vi "IMAQdx Acquisition Template (Host)RT-8output.vi"() -> ()   [LabVIEW 2016]
uses:
  <vilib>/userdefined/High Color/IMAQdx.ctl
  <vilib>/FPGAPlugInAG/roboRIO/niLvFpga_Open_roboRIO.vi
  <vilib>/rvi/interface/common/dynamic/niFpgaDynamicAddResources.vi
  <vilib>/FPGAPlugInAG/Dynamic/niLvFpga_Download_Dynamic.vi
  <vilib>/FPGAPlugInAG/Dynamic/niLvFpga_Run_Dynamic.vi
  <vilib>/Utility/error.llb/Error Cluster From Error Code.vi
  <vilib>/rvi/errors/niLvFpgaAdjustHostInterfaceError.vi
  <vilib>/rvi/interface/common/niFpgaWaitOnOcc.vi
  <vilib>/vision/EDVR.llb/IMAQ ImageToEDVR 2D U32.vi
  <vilib>/FPGAPlugInAG/Dynamic/niLvFpga_Close_Dynamic.vi
  <vilib>/rvi/interface/nirviOpenFPGA/nirviOpenFPGA.xnode
  FPGA Bitfiles/ImageProcessingw_FPGATarget_ImageProcessingw_Z23Lc7CsNwk.lvbitx
  <vilib>/rvi/interface/nirviMethod/nirviMethod.xnode
  <vilib>/rvi/interface/nirviReadWriteControl/nirviReadWriteControl.xnode
  <vilib>/rvi/interface/nirviCloseFPGA/nirviCloseFPGA.xnode
  <vilib>/vision/driver/NI_Vision_Acquisition_Software.lvlib
  <resource>/objmgr/imaqdx.rc
  <vilib>/rvi/interface/Simulation/niFpgaSimulationCallBeginRW.vi
  <vilib>/rvi/errors/niLvFpgaMergeErrorWithErrorCode.vi
  <vilib>/FPGAPlugInAG/Dynamic/niLvFpga_ReadFifo_Dynamic.vi
  <vilib>/FPGAPlugInAG/Dynamic/niLvFpga_ConfigureFifo_Dynamic.vi
  <vilib>/FPGAPlugInAG/Dynamic/niLvFpga_StartFifo_Dynamic.vi
  NiFpgaLv.dll
  <vilib>/FPGAPlugInAG/Dynamic/niLvFpga_WriteFifo_Dynamic.vi
panel:
  out "RecGaussian2?":bool
  out "RecGaussian1?":bool
  out "Error Out 2":errorcluster
  in  "Stop":bool
  in  "Maximum Pixels per Write":u32=261244
  out "dePixelCount":u32
  out "AllPixelCount":u32
  out "error out 2":errorcluster
  in  "Camera":T1="cam0"
  # "Overview: Demonstrates how to acquire an image from a camera using the IMAQdx API, transfer the image to a FPGA target for processing, and retrieve the processed image for display or further processing on the host.\nRequirements:\n- LabVIEW FPGA\n- Vision Acquisition Software\n- Vision Development Module\nInstructions:\n1. Select a Camera\n2. Run the VI."
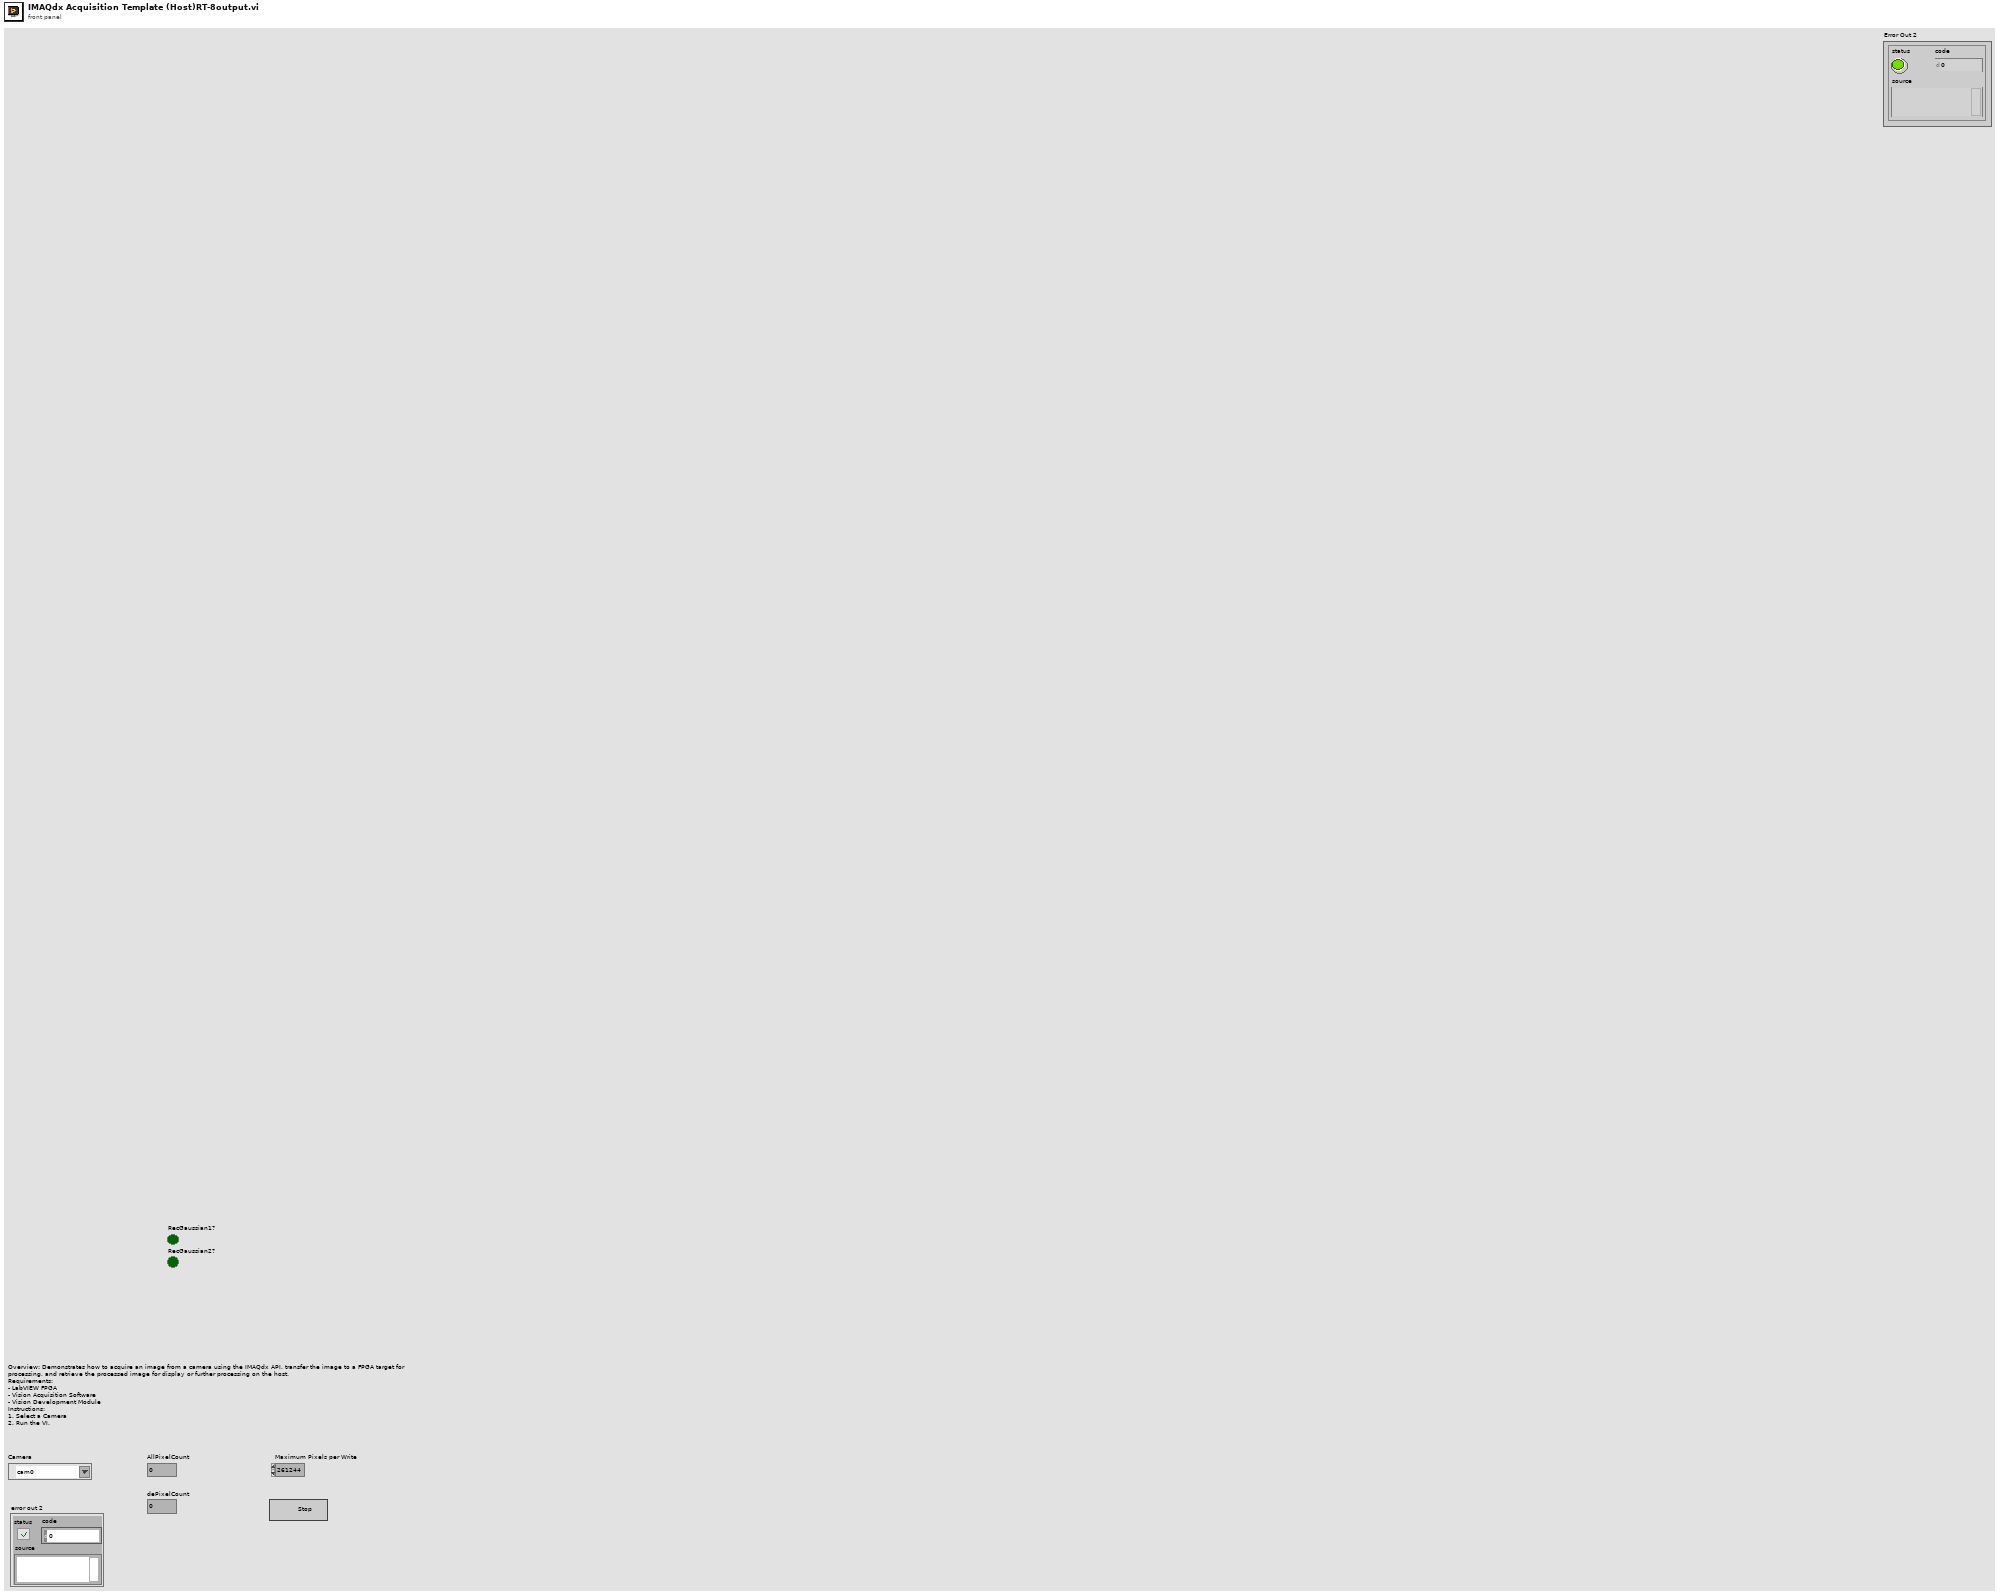
[diagram p1: front panel]
types:
  T1 = typedef "IMAQdx.ctl" = refnum<k21>
  T2 = typedef "Image Type" = u32
  T3 = typedef "IMAQ Image.ctl" = refnum<image>
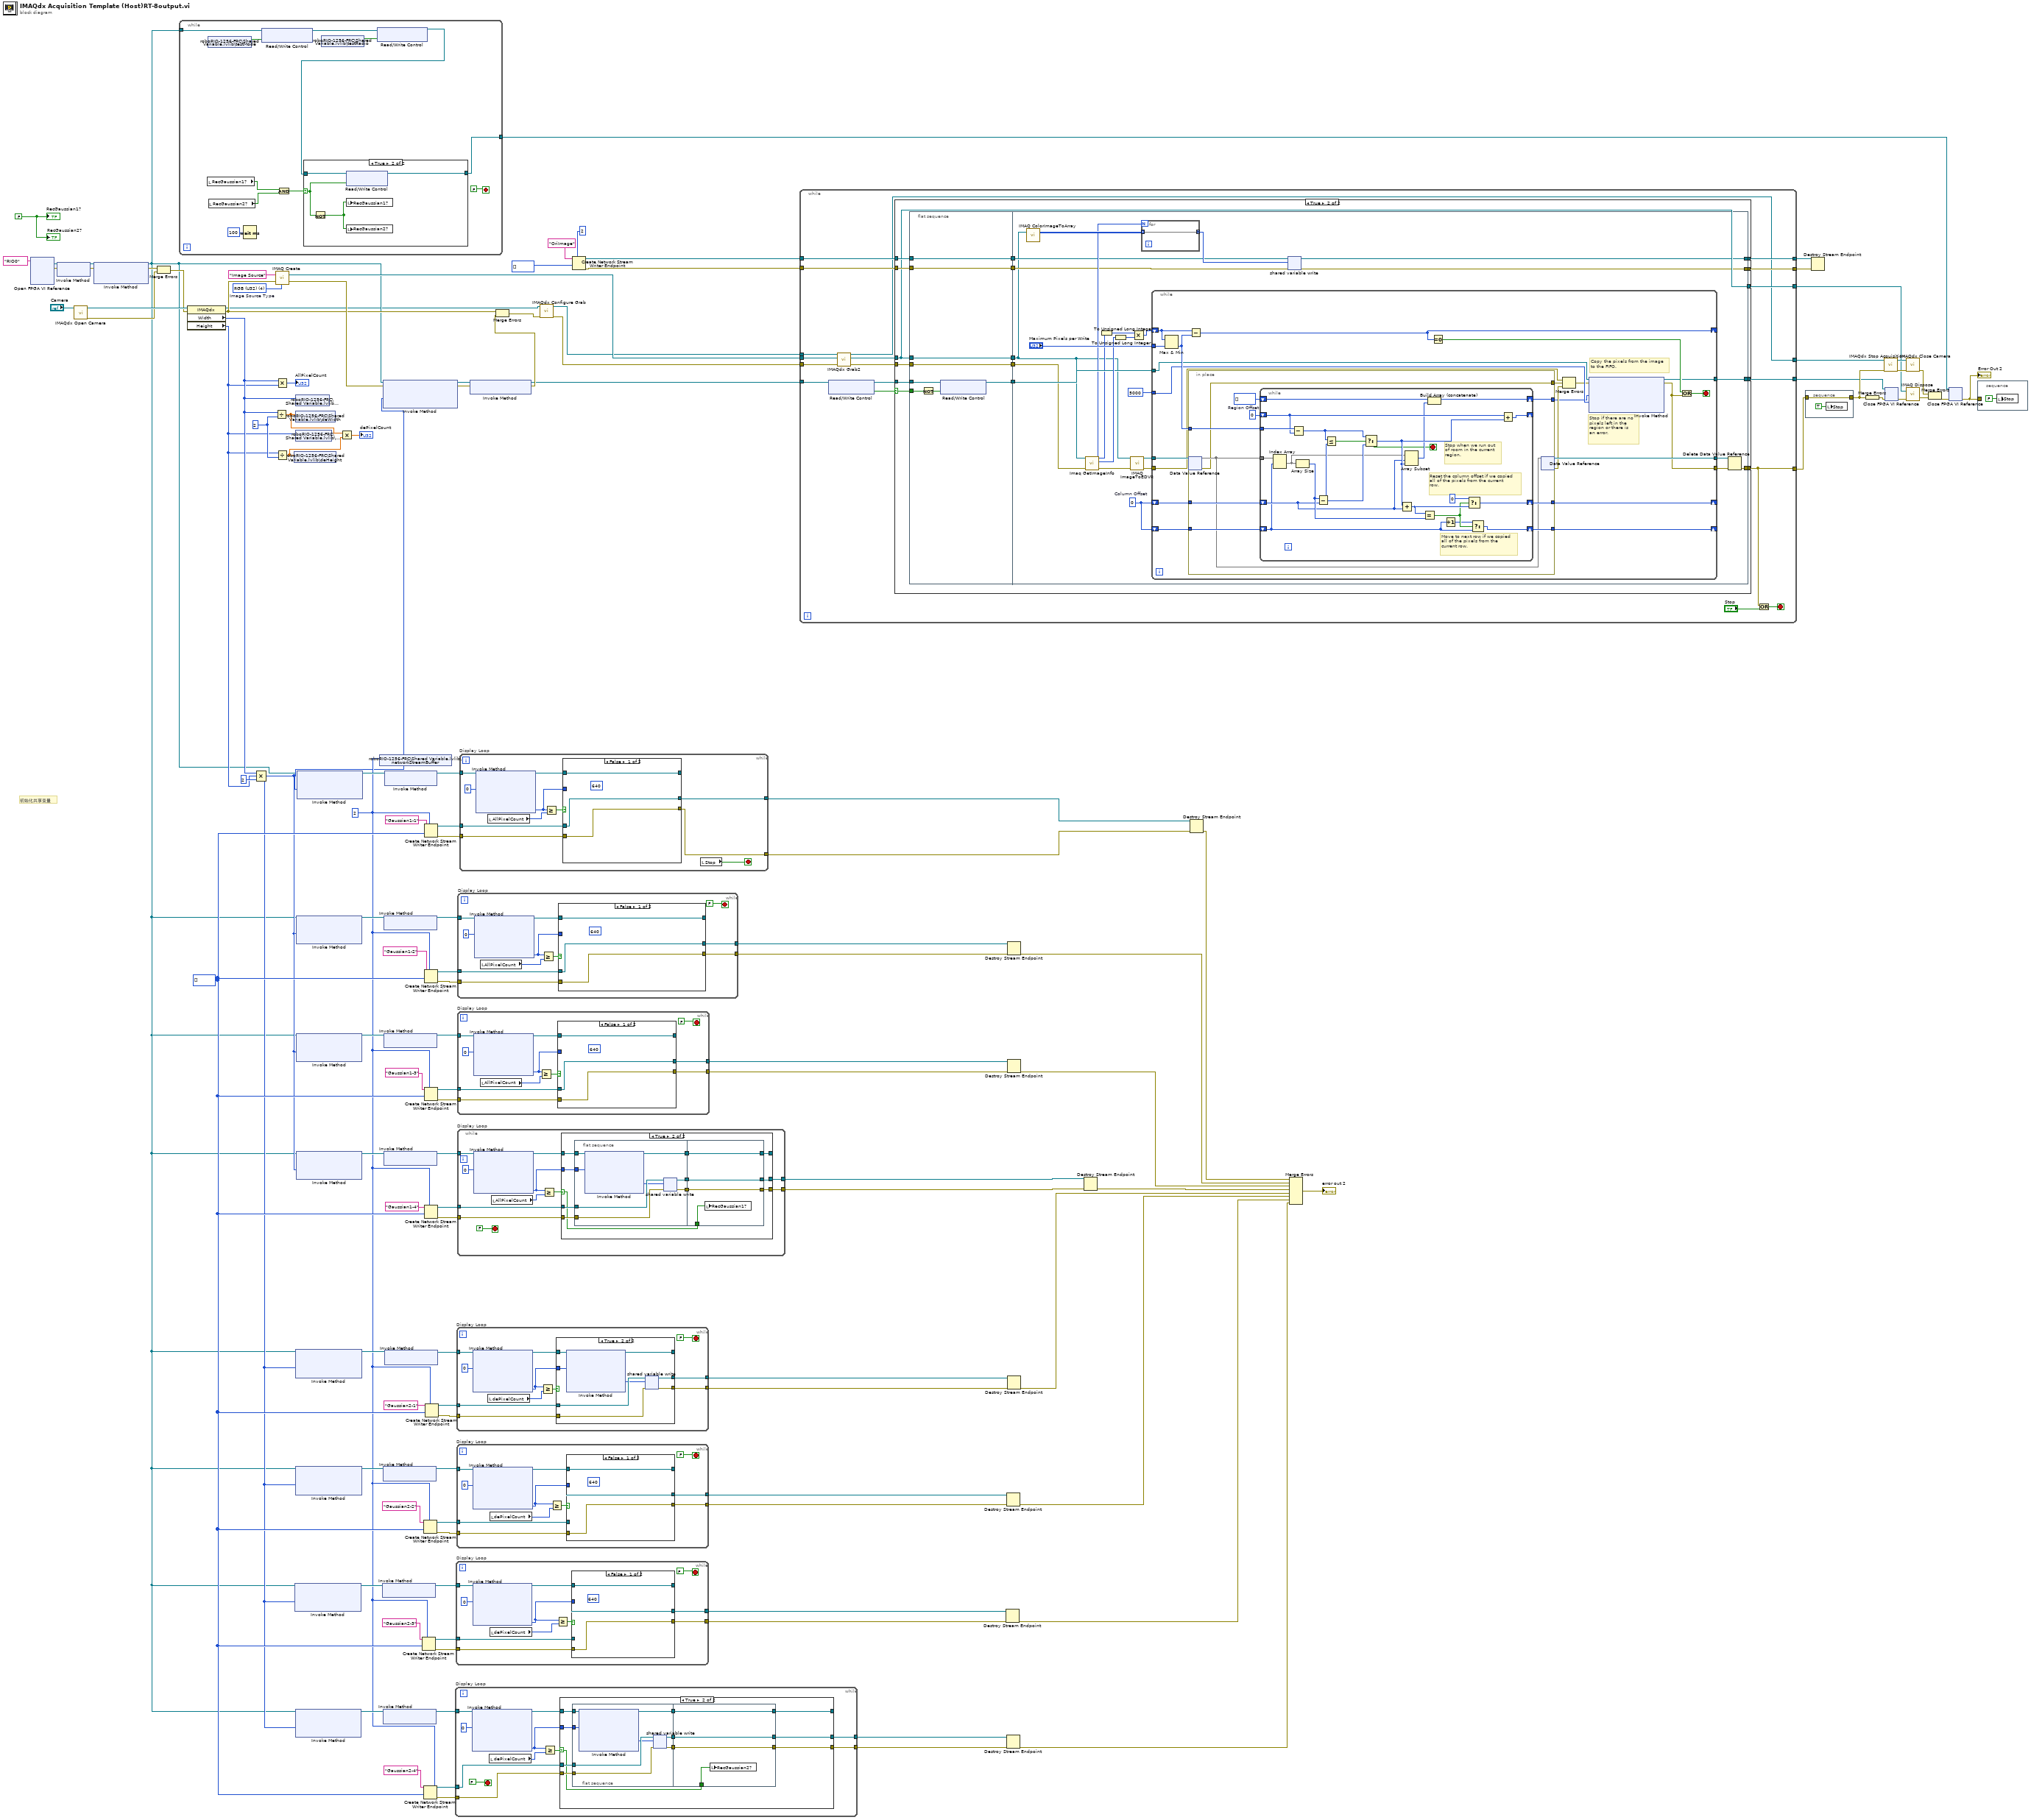
[diagram p0: block diagram]
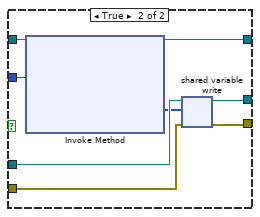
[diagram p4: hidden frame]
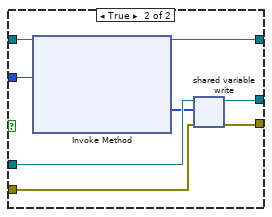
[diagram p5: hidden frame]
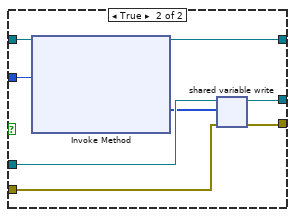
[diagram p9: hidden frame]
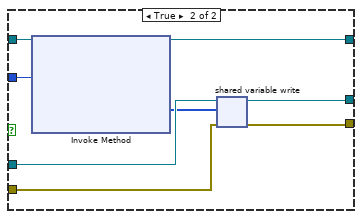
[diagram p10: hidden frame]
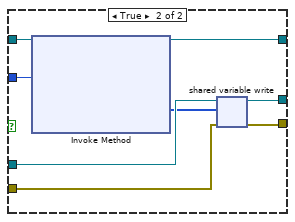
[diagram p11: hidden frame]
diagram:
  w1 = FALSE
  w42 = u32 2 ("y")
  w51 = i32[] []
  w48 = 2 ("writer buffer size")
  w111 = T2 4 items=["Grayscale (U8)", "Grayscale (I16)", "Grayscale (SGL)", "Complex (CSG)", "RGB (U32)", "HSL (U32)", "RGB (U64)", "Grayscale (U16)"]  # Image Source Type
  # "初始化共享变量"
  n1 = xnode "Open FPGA VI Reference"("resource name"=tag "RIO0") -> ("FPGA VI Reference Out"=w118:refnum<k20>, "error out"=w119:errorcluster)  [unwired: 1 in]
  n2 = xnode "Invoke Method"("FPGA VI Reference In"=w118, "error in"=w119) -> ("FPGA VI Reference Out"=w121:refnum<k20>, "error out"=w120:errorcluster)
  n3 = call <vilib>:"IMAQdx Open Camera.vi"("Session In"="Camera") -> ("error out"=w113:errorcluster, "Session Out"=w114:T1)  [unwired: 9 in]
  n4 = xnode "Invoke Method"("FPGA VI Reference In"=w121, "error in"=w120) -> ("FPGA VI Reference Out"=w6:refnum<k20>, "error out"=w115:errorcluster)  [unwired: 1 in]
  n5 = Merge Errors(w115, w113) -> (w112:errorcluster)
  n6 = while {
    tunnel: w6 -> [w128]
    tunnel: [w123] -> w9
    stop <- FALSE stop-if-true
    n7 = local read "RecGaussian1?"() -> (w132:bool)
    n8 = shared-variable "roboRIO-1256-FRC\\Shared Variable.lvlib\\testMode"() -> (w127:bool)  [unwired: 1 in, 1 out]
    n9 = local read "RecGaussian2?"() -> (w131:bool)
    n10 = Wait (ms)(milliseconds to wait=u32 100) -> ()  [unwired: 1 out]
    n11 = xnode "Read/Write Control"("FPGA VI Reference In"=w128, "Mode LED Status"=w127) -> ("FPGA VI Reference Out"=w126:refnum<k20>)  [unwired: 1 in, 1 out]
    n12 = And(x=w132, y=w131) -> (x .and. y?=w130:bool)
    n13 = shared-variable "roboRIO-1256-FRC\\Shared Variable.lvlib\\testRadio"() -> (w125:bool)  [unwired: 1 in, 1 out]
    n14 = xnode "Read/Write Control"("FPGA VI Reference In"=w126, "Radio LED Status"=w125) -> ("FPGA VI Reference Out"=w124:refnum<k20>)  [unwired: 1 in, 1 out]
    n15 = case shown="True" w130 {
      selector: w130 -> [_ w136]
      tunnel: w124 -> [w134 w138]
      tunnel: [w134 w137] -> w123
      frame False {
      }
      frame True {
        n16 = Not(x=w136) -> (.not. x?=w135:bool)
        n17 = xnode "Read/Write Control"("FPGA VI Reference In"=w138, "StartOfImage"=w136) -> ("FPGA VI Reference Out"=w137:refnum<k20>)  [unwired: 1 in, 1 out]
        n18 = local write "RecGaussian1?"(w135) -> ()
        n19 = local write "RecGaussian2?"(w135) -> ()
      }
    }
  }
  n20 = property class="IMAQdx"(reference=w114, error in=w112) -> (reference out=w5:T1, error out=w31:errorcluster, "Width"=w41:u32, "Height"=w40:u32)
  n21 = Compound Arithmetic op=MULTIPLY(w41, w40, u32 2 ("value")) -> (w35:u32)
  n22 = Divide(x=w41, y=w42) -> (x/y=w37:dbl)
  n23 = call "IMAQ Create"("Image Name"="Image Source", "Image Type"=w111, "error in (no error)"=w31) -> ("New Image"=w7:T3, "error out"=w34:errorcluster)  [unwired: 2 in]
  n24 = Multiply(x=w41, y=w40) -> (x*y=→"AllPixelCount":u32)
  n25 = Divide(x=w40, y=w42) -> (x/y=w36:dbl)
  n26 = shared-variable "roboRIO-1256-FRC\\Shared Variable.lvlib\\deHeight"(w36) -> ()  [unwired: 1 in, 1 out]
  n27 = xnode "Invoke Method"("FPGA VI Reference In"=w6, "Requested Depth"=w35) -> ("FPGA VI Reference Out"=w56:refnum<k20>)  [unwired: 1 in, 2 out]
  n28 = shared-variable "roboRIO-1256-FRC\\Shared Variable.lvlib\\Width"(w41) -> ()  [unwired: 1 in, 1 out]
  n29 = shared-variable "roboRIO-1256-FRC\\Shared Variable.lvlib\\deWidth"(w37) -> ()  [unwired: 1 in, 1 out]
  n30 = xnode "Invoke Method"("FPGA VI Reference In"=w6, "Requested Depth"=w35) -> ("FPGA VI Reference Out"=w79:refnum<k20>)  [unwired: 1 in, 2 out]
  n31 = shared-variable "roboRIO-1256-FRC\\Shared Variable.lvlib\\Height"(w40) -> ()  [unwired: 1 in, 1 out]
  n32 = xnode "Invoke Method"("FPGA VI Reference In"=w6, "Requested Depth"=w35) -> ("FPGA VI Reference Out"=w50:refnum<k20>)  [unwired: 1 in, 2 out]
  n33 = xnode "Invoke Method"("FPGA VI Reference In"=w6, "Requested Depth"=w35) -> ("FPGA VI Reference Out"=w61:refnum<k20>)  [unwired: 1 in, 2 out]
  n34 = xnode "Invoke Method"("FPGA VI Reference In"=w6, "Requested Depth"=w35) -> ("FPGA VI Reference Out"=w94:refnum<k20>)  [unwired: 1 in, 2 out]
  n35 = xnode "Invoke Method"("FPGA VI Reference In"=w6, "Requested Depth"=w35) -> ("FPGA VI Reference Out"=w91:refnum<k20>)  [unwired: 1 in, 2 out]
  n36 = xnode "Invoke Method"("FPGA VI Reference In"=w6, "Requested Depth"=w35) -> ("FPGA VI Reference Out"=w73:refnum<k20>)  [unwired: 1 in, 2 out]
  n37 = xnode "Invoke Method"("FPGA VI Reference In"=w6, "Requested Depth"=w35) -> ("FPGA VI Reference Out"=w110:refnum<k20>)  [unwired: 1 in, 2 out]
  n38 = Multiply(x=w37, y=w36) -> (x*y=→"dePixelCount":dbl)
  n39 = shared-variable "roboRIO-1256-FRC\\Shared Variable.lvlib\\networkStreamBuffer"(w48) -> ()  [unwired: 1 in, 1 out]
  n40 = xnode "Invoke Method"("FPGA VI Reference In"=w56) -> ("FPGA VI Reference Out"=w57:refnum<k20>)  [unwired: 1 in, 1 out]
  n41 = xnode "Invoke Method"("FPGA VI Reference In"=w6, "error in"=w34, "Requested Depth"=w35) -> ("FPGA VI Reference Out"=w33:refnum<k20>, "error out"=w32:errorcluster)  [unwired: 1 out]
  n42 = xnode "Invoke Method"("FPGA VI Reference In"=w79) -> ("FPGA VI Reference Out"=w78:refnum<k20>)  [unwired: 1 in, 1 out]
  n43 = xnode "Invoke Method"("FPGA VI Reference In"=w61) -> ("FPGA VI Reference Out"=w60:refnum<k20>)  [unwired: 1 in, 1 out]
  n44 = xnode "Invoke Method"("FPGA VI Reference In"=w94) -> ("FPGA VI Reference Out"=w93:refnum<k20>)  [unwired: 1 in, 1 out]
  n45 = xnode "Invoke Method"("FPGA VI Reference In"=w91) -> ("FPGA VI Reference Out"=w92:refnum<k20>)  [unwired: 1 in, 1 out]
  n46 = xnode "Invoke Method"("FPGA VI Reference In"=w73) -> ("FPGA VI Reference Out"=w72:refnum<k20>)  [unwired: 1 in, 1 out]
  n47 = xnode "Invoke Method"("FPGA VI Reference In"=w110) -> ("FPGA VI Reference Out"=w109:refnum<k20>)  [unwired: 1 in, 1 out]
  n48 = xnode "Invoke Method"("FPGA VI Reference In"=w50) -> ("FPGA VI Reference Out"=w49:refnum<k20>)  [unwired: 1 in, 1 out]
  n49 = Create Network Stream Writer Endpoint(7:w48, 9:w51, 11:"Gaussian2-3" ("writer name")) -> (0:w55:errorcluster, 3:w54:refnum<k21>)  [unwired: 4 in]
  n50 = Create Network Stream Writer Endpoint(7:w48, 9:w51, 11:"Gaussian2-4" ("writer name")) -> (0:w80:errorcluster, 3:w81:refnum<k21>)  [unwired: 4 in]
  n51 = Create Network Stream Writer Endpoint(7:w48, 9:w51, 11:"Gaussian2-2" ("writer name")) -> (0:w62:errorcluster, 3:w63:refnum<k21>)  [unwired: 4 in]
  n52 = Create Network Stream Writer Endpoint(7:w48, 9:w51, 11:"Gaussian1-1" ("writer name")) -> (0:w104:errorcluster, 3:w103:refnum<k21>)  [unwired: 4 in]
  n53 = Create Network Stream Writer Endpoint(7:w48, 9:w51, 11:"Gaussian1-2" ("writer name")) -> (0:w95:errorcluster, 3:w96:refnum<k21>)  [unwired: 4 in]
  n54 = Create Network Stream Writer Endpoint(7:w48, 9:w51, 11:"Gaussian1-3" ("writer name")) -> (0:w90:errorcluster, 3:w89:refnum<k21>)  [unwired: 4 in]
  n55 = Create Network Stream Writer Endpoint(7:w48, 9:w51, 11:"Gaussian1-4" ("writer name")) -> (0:w74:errorcluster, 3:w75:refnum<k21>)  [unwired: 4 in]
  n56 = Create Network Stream Writer Endpoint(7:w48, 9:w51, 11:"Gaussian2-1" ("writer name")) -> (0:w69:errorcluster, 3:w68:refnum<k21>)  [unwired: 4 in]
  n57 = while "Display Loop" {
    tunnel: [w149] -> w84
    tunnel: w80 -> [w148]
    tunnel: w81 -> [w147]
    tunnel: [w143] -> w83
    tunnel: w78 -> [w142]
    stop <- FALSE stop-if-true
    n58 = xnode "Invoke Method"("FPGA VI Reference In"=w142, "Number of Elements"=u32 0) -> ("FPGA VI Reference Out"=w145:refnum<k20>, "Elements Remaining"=w139:u32)  [unwired: 2 in, 2 out]
    n59 = local read "dePixelCount"() -> (w140:u32)
    n60 = Greater Or Equal?(x=w139, y=w140) -> (x >= y?=w141:bool)
    n61 = case shown="True" w141 {
      selector: w141 -> [_ w153]
      tunnel: w145 -> [w150 w163]
      tunnel: [w152 w162] -> w149
      tunnel: w148 -> [w151 w161]
      tunnel: w147 -> [w152 w160]
      tunnel: [w151 w159] -> w143
      tunnel: [w150 w158] -> _
      tunnel: w139 -> [_ w157]
      frame False {
      }
      frame True {
        n62 = flat-sequence {
          tunnel: w163 -> [w171]
          tunnel: w161 -> [w169]
          tunnel: w160 -> [w168]
          tunnel: w157 -> [w164]
          tunnel: [w170] -> w156
          tunnel: [w167] -> w155
          tunnel: [w166] -> w154
          tunnel: [w173] -> w158
          tunnel: [w174] -> w159
          tunnel: [w175] -> w162
          tunnel: w156 -> [w175]
          tunnel: w155 -> [w174]
          tunnel: w154 -> [w173]
          tunnel: w153 -> [w172]
          frame #0 {
            n63 = xnode "Invoke Method"("FPGA VI Reference In"=w171, "Number of Elements"=w164) -> ("FPGA VI Reference Out"=w166:refnum<k20>, "Data"=w165:u8[])  [unwired: 2 in, 2 out]
            n64 = shared-variable-write(w168, w169, w165) -> (w170:refnum<k21>, w167:errorcluster)  [unwired: 1 in, 1 out]
          }
          frame #1 {
            n65 = local write "RecGaussian2?"(w172) -> ()
          }
        }
      }
    }
  }
  n66 = while "Display Loop" {
    tunnel: [w186] -> w52
    tunnel: w55 -> [w185]
    tunnel: w54 -> [w184]
    tunnel: [w180] -> w53
    tunnel: w57 -> [w179]
    stop <- FALSE stop-if-true
    (unwired) u32 640 ("Number of Elements")
    n67 = xnode "Invoke Method"("FPGA VI Reference In"=w179, "Number of Elements"=u32 0) -> ("FPGA VI Reference Out"=w182:refnum<k20>, "Elements Remaining"=w176:u32)  [unwired: 2 in, 2 out]
    n68 = local read "dePixelCount"() -> (w177:u32)
    n69 = Greater Or Equal?(x=w176, y=w177) -> (x >= y?=w178:bool)
    n70 = case shown="False" w178 {
      tunnel: w182 -> [w187 w197]
      tunnel: [w189 w196] -> w186
      tunnel: w185 -> [w188 w195]
      tunnel: w184 -> [w189 w194]
      tunnel: [w188 w193] -> w180
      tunnel: [w187 w191] -> _
      tunnel: w176 -> [_ w190]
      frame False {
      }
      frame True {
        n71 = xnode "Invoke Method"("FPGA VI Reference In"=w197, "Number of Elements"=w190) -> ("FPGA VI Reference Out"=w191:refnum<k20>, "Data"=w192:u8[])  [unwired: 2 in, 2 out]
        n72 = shared-variable-write(w194, w195, w192) -> (w196:refnum<k21>, w193:errorcluster)  [unwired: 1 in, 1 out]
      }
    }
  }
  n73 = while "Display Loop" {
    tunnel: [w208] -> w66
    tunnel: w69 -> [w207]
    tunnel: w68 -> [w206]
    tunnel: [w202] -> w67
    tunnel: w49 -> [w201]
    stop <- FALSE stop-if-true
    (unwired) u32 640 ("Number of Elements")
    n74 = xnode "Invoke Method"("FPGA VI Reference In"=w201, "Number of Elements"=u32 0) -> ("FPGA VI Reference Out"=w204:refnum<k20>, "Elements Remaining"=w198:u32)  [unwired: 2 in, 2 out]
    n75 = local read "dePixelCount"() -> (w199:u32)
    n76 = Greater Or Equal?(x=w198, y=w199) -> (x >= y?=w200:bool)
    n77 = case shown="True" w200 {
      tunnel: w204 -> [w209 w219]
      tunnel: [w211 w218] -> w208
      tunnel: w207 -> [w210 w217]
      tunnel: w206 -> [w211 w216]
      tunnel: [w210 w215] -> w202
      tunnel: [w209 w213] -> _
      tunnel: w198 -> [_ w212]
      frame False {
      }
      frame True {
        n78 = xnode "Invoke Method"("FPGA VI Reference In"=w219, "Number of Elements"=w212) -> ("FPGA VI Reference Out"=w213:refnum<k20>, "Data"=w214:u8[])  [unwired: 2 in, 2 out]
        n79 = shared-variable-write(w216, w217, w214) -> (w218:refnum<k21>, w215:errorcluster)  [unwired: 1 in, 1 out]
      }
    }
  }
  n80 = while "Display Loop" {
    tunnel: [w230] -> w65
    tunnel: w62 -> [w229]
    tunnel: w63 -> [w228]
    tunnel: [w224] -> w64
    tunnel: w60 -> [w223]
    stop <- FALSE stop-if-true
    (unwired) u32 640 ("Number of Elements")
    n81 = xnode "Invoke Method"("FPGA VI Reference In"=w223, "Number of Elements"=u32 0) -> ("FPGA VI Reference Out"=w226:refnum<k20>, "Elements Remaining"=w220:u32)  [unwired: 2 in, 2 out]
    n82 = local read "dePixelCount"() -> (w221:u32)
    n83 = Greater Or Equal?(x=w220, y=w221) -> (x >= y?=w222:bool)
    n84 = case shown="False" w222 {
      tunnel: w226 -> [w231 w241]
      tunnel: [w233 w240] -> w230
      tunnel: w229 -> [w232 w239]
      tunnel: w228 -> [w233 w238]
      tunnel: [w232 w237] -> w224
      tunnel: [w231 w235] -> _
      tunnel: w220 -> [_ w234]
      frame False {
      }
      frame True {
        n85 = xnode "Invoke Method"("FPGA VI Reference In"=w241, "Number of Elements"=w234) -> ("FPGA VI Reference Out"=w235:refnum<k20>, "Data"=w236:u8[])  [unwired: 2 in, 2 out]
        n86 = shared-variable-write(w238, w239, w236) -> (w240:refnum<k21>, w237:errorcluster)  [unwired: 1 in, 1 out]
      }
    }
  }
  n87 = while "Display Loop" {
    tunnel: [w252] -> w86
    tunnel: w90 -> [w251]
    tunnel: w89 -> [w250]
    tunnel: [w246] -> w87
    tunnel: w92 -> [w245]
    stop <- FALSE stop-if-true
    (unwired) u32 640 ("Number of Elements")
    n88 = xnode "Invoke Method"("FPGA VI Reference In"=w245, "Number of Elements"=u32 0) -> ("FPGA VI Reference Out"=w248:refnum<k20>, "Elements Remaining"=w242:u32)  [unwired: 2 in, 2 out]
    n89 = local read "AllPixelCount"() -> (w244:u32)
    n90 = Greater Or Equal?(x=w242, y=w244) -> (x >= y?=w243:bool)
    n91 = case shown="False" w243 {
      tunnel: w248 -> [w253 w263]
      tunnel: [w255 w262] -> w252
      tunnel: w251 -> [w254 w261]
      tunnel: w250 -> [w255 w260]
      tunnel: [w254 w259] -> w246
      tunnel: [w253 w257] -> _
      tunnel: w242 -> [_ w256]
      frame False {
      }
      frame True {
        n92 = xnode "Invoke Method"("FPGA VI Reference In"=w263, "Number of Elements"=w256) -> ("FPGA VI Reference Out"=w257:refnum<k20>, "Data"=w258:u8[])  [unwired: 2 in, 2 out]
        n93 = shared-variable-write(w260, w261, w258) -> (w262:refnum<k21>, w259:errorcluster)  [unwired: 1 in, 1 out]
      }
    }
  }
  n94 = while "Display Loop" {
    tunnel: [w274] -> w77
    tunnel: w74 -> [w273]
    tunnel: w75 -> [w272]
    tunnel: [w268] -> w76
    tunnel: w72 -> [w267]
    stop <- FALSE stop-if-true
    n95 = xnode "Invoke Method"("FPGA VI Reference In"=w267, "Number of Elements"=u32 0) -> ("FPGA VI Reference Out"=w270:refnum<k20>, "Elements Remaining"=w264:u32)  [unwired: 2 in, 2 out]
    n96 = local read "AllPixelCount"() -> (w266:u32)
    n97 = Greater Or Equal?(x=w264, y=w266) -> (x >= y?=w265:bool)
    n98 = case shown="True" w265 {
      selector: w265 -> [_ w278]
      tunnel: w270 -> [w275 w283]
      tunnel: [w277 w288] -> w274
      tunnel: w273 -> [w276 w287]
      tunnel: w272 -> [w277 w286]
      tunnel: [w276 w285] -> w268
      tunnel: [w275 w284] -> _
      tunnel: w264 -> [_ w282]
      frame False {
      }
      frame True {
        n99 = flat-sequence {
          tunnel: w287 -> [w295]
          tunnel: w286 -> [w294]
          tunnel: w283 -> [w290]
          tunnel: w282 -> [w289]
          tunnel: [w296] -> w281
          tunnel: [w293] -> w280
          tunnel: [w292] -> w279
          tunnel: [w298] -> w284
          tunnel: [w299] -> w285
          tunnel: [w300] -> w288
          tunnel: w281 -> [w300]
          tunnel: w280 -> [w299]
          tunnel: w279 -> [w298]
          tunnel: w278 -> [w297]
          frame #0 {
            n100 = xnode "Invoke Method"("FPGA VI Reference In"=w290, "Number of Elements"=w289) -> ("FPGA VI Reference Out"=w292:refnum<k20>, "Data"=w291:u8[])  [unwired: 2 in, 2 out]
            n101 = shared-variable-write(w294, w295, w291) -> (w296:refnum<k21>, w293:errorcluster)  [unwired: 1 in, 1 out]
          }
          frame #1 {
            n102 = local write "RecGaussian1?"(w297) -> ()
          }
        }
      }
    }
  }
  n103 = while "Display Loop" {
    tunnel: [w311] -> w102
    tunnel: w95 -> [w310]
    tunnel: w96 -> [w309]
    tunnel: [w305] -> w101
    tunnel: w93 -> [w304]
    stop <- FALSE stop-if-true
    (unwired) u32 640 ("Number of Elements")
    n104 = xnode "Invoke Method"("FPGA VI Reference In"=w304, "Number of Elements"=u32 0) -> ("FPGA VI Reference Out"=w307:refnum<k20>, "Elements Remaining"=w301:u32)  [unwired: 2 in, 2 out]
    n105 = local read "AllPixelCount"() -> (w303:u32)
    n106 = Greater Or Equal?(x=w301, y=w303) -> (x >= y?=w302:bool)
    n107 = case shown="False" w302 {
      tunnel: w307 -> [w312 w322]
      tunnel: [w314 w321] -> w311
      tunnel: w310 -> [w313 w320]
      tunnel: w309 -> [w314 w319]
      tunnel: [w313 w318] -> w305
      tunnel: [w312 w316] -> _
      tunnel: w301 -> [_ w315]
      frame False {
      }
      frame True {
        n108 = xnode "Invoke Method"("FPGA VI Reference In"=w322, "Number of Elements"=w315) -> ("FPGA VI Reference Out"=w316:refnum<k20>, "Data"=w317:u8[])  [unwired: 2 in, 2 out]
        n109 = shared-variable-write(w319, w320, w317) -> (w321:refnum<k21>, w318:errorcluster)  [unwired: 1 in, 1 out]
      }
    }
  }
  n110 = while "Display Loop" {
    tunnel: w109 -> [w327]
    tunnel: [w329] -> w106
    tunnel: [w332] -> w105
    tunnel: w104 -> [w331]
    tunnel: w103 -> [w330]
    stop <- w333 stop-if-true
    (unwired) u32 640 ("Number of Elements")
    n111 = xnode "Invoke Method"("FPGA VI Reference In"=w327, "Number of Elements"=u32 0) -> ("FPGA VI Reference Out"=w326:refnum<k20>, "Elements Remaining"=w323:u32)  [unwired: 2 in, 2 out]
    n112 = local read "AllPixelCount"() -> (w324:u32)
    n113 = Greater Or Equal?(x=w323, y=w324) -> (x >= y?=w325:bool)
    n114 = case shown="False" w325 {
      tunnel: w326 -> [w334 w344]
      tunnel: [w336 w343] -> w332
      tunnel: w331 -> [w335 w342]
      tunnel: w330 -> [w336 w341]
      tunnel: [w335 w340] -> w329
      tunnel: [w334 w338] -> _
      tunnel: w323 -> [_ w337]
      frame False {
      }
      frame True {
        n115 = xnode "Invoke Method"("FPGA VI Reference In"=w344, "Number of Elements"=w337) -> ("FPGA VI Reference Out"=w338:refnum<k20>, "Data"=w339:u8[])  [unwired: 2 in, 2 out]
        n116 = shared-variable-write(w341, w342, w339) -> (w343:refnum<k21>, w340:errorcluster)  [unwired: 1 in, 1 out]
      }
    }
    n117 = local read "Stop"() -> (w333:bool)
  }
  n118 = xnode "Invoke Method"("FPGA VI Reference In"=w33, "error in"=w32) -> ("FPGA VI Reference Out"=w8:refnum<k20>, "error out"=w30:errorcluster)
  n119 = Merge Errors(w31, w30) -> (w4:errorcluster)
  n120 = call <vilib>:"IMAQdx Configure Grab.vi"("error in"=w4, "Session In"=w5) -> ("error out"=w2:errorcluster, "Session Out"=w3:T1)  [unwired: 8 in]
  n121 = Create Network Stream Writer Endpoint(7:2 ("writer buffer size"), 9:i32[] [], 11:"OriImage" ("writer name")) -> (0:w23:errorcluster, 3:w24:refnum<k21>)  [unwired: 4 in]
  n122 = while {
    tunnel: [w360] -> w29
    tunnel: [w359] -> w28
    tunnel: w24 -> [w358]
    tunnel: w23 -> [w357]
    tunnel: [w350] -> w13
    tunnel: w3 -> [w347]
    tunnel: w7 -> [w346]
    tunnel: w2 -> [w345]
    tunnel: w8 -> [w353]
    tunnel: [w356] -> w11
    tunnel: [w355] -> w12
    tunnel: [w354] -> w10
    stop <- w361 stop-if-true
    n123 = xnode "Read/Write Control"("FPGA VI Reference In"=w353) -> ("FPGA VI Reference Out"=w352:refnum<k20>, "CanSendImage"=w351:bool)  [unwired: 1 in, 1 out]
    n124 = call <vilib>:"IMAQdx Grab2.vi"("error in"=w345, "Image In"=w346, "Session In"=w347) -> ("error out"=w348:errorcluster, "Image Out"=w349:T3, "Session Out"=w350:T1)  [unwired: 5 in, 1 out]
    n125 = case shown="True" w351 {
      selector: w351 -> [_ w368]
      tunnel: w352 -> [w364 w382]
      tunnel: w349 -> [w365 w374]
      tunnel: [w363 w381] -> w356
      tunnel: [w367 w380] -> w360
      tunnel: [w366 w379] -> w359
      tunnel: w358 -> [w367 w378]
      tunnel: w357 -> [w366 w377]
      tunnel: w348 -> [w363 w376]
      tunnel: [w364 w375] -> w355
      tunnel: [w365 w374] -> w354
      frame False {
      }
      frame True {
        n126 = flat-sequence {
          tunnel: w374 -> [w387]
          tunnel: w376 -> [w388]
          tunnel: w377 -> [w389]
          tunnel: w378 -> [w390]
          tunnel: w382 -> [w385]
          tunnel: [w384] -> w373
          tunnel: [w390] -> w372
          tunnel: [w389] -> w371
          tunnel: [w388] -> w370
          tunnel: [w387] -> w369
          tunnel: w368 -> [w386]
          tunnel: [w399] -> w381
          tunnel: [w397] -> w380
          tunnel: [w396] -> w379
          tunnel: [w392] -> w375
          tunnel: w373 -> [w402]
          tunnel: w372 -> [w395]
          tunnel: w371 -> [w394]
          tunnel: w370 -> [w393]
          tunnel: w369 -> [w391]
          frame #0 {
            n127 = Not(x=w386) -> (.not. x?=w383:bool)
            n128 = xnode "Read/Write Control"("FPGA VI Reference In"=w385, "CanSendImage"=w383) -> ("FPGA VI Reference Out"=w384:refnum<k20>)  [unwired: 1 in, 1 out]
          }
          frame #1 {
            w404 = u32 0  # Column Offset
            n129 = call "IMAQ ColorImageToArray"("Image"=w391) -> ("Image Pixels (U32)"=w401:u32[][])  [unwired: 3 in, 2 out]
            n130 = call "Imaq GetImageInfo"("error in (no error)"=w393, "Image"=w391) -> ("error out"=w410:errorcluster, "Y Resolution"=w411:i32, "X Resolution"=w400:i32)  [unwired: 2 in, 5 out]
            n131 = To Unsigned Long Integer(number=w400) -> (unsigned 32bit integer=w413:u32)
            n132 = To Unsigned Long Integer(number=w411) -> (unsigned 32bit integer=w414:u32)
            n133 = call-poly <vilib>:"IMAQ ImageToEDVR.vi"("error out"=w410, "Image"=w391) -> ("error out"=w408:errorcluster, "EDVR 2D U32"=w409:refnum<data-value>)  [unwired: 7 in, 1 out]
            n134 = Multiply(x=w413, y=w414) -> (x*y=w405:u32)
            n135 = for {
              N: w400 -> [_]
              tunnel: w401 -> [w415] mode=indexing
              tunnel: [w415] -> w398 mode=concatenating
            }
            n136 = while {
              shift-right: [w430] -> _
              shift-left: w405 -> [w427]
              tunnel: w409 -> [w436]
              shift-right: [w432] -> _
              shift-left: w404 -> [w434]
              shift-right: [w435] -> _
              shift-left: w404 -> [w433]
              tunnel: w402 -> [w421]
              tunnel: [w431] -> w407
              tunnel: [w419] -> w406
              tunnel: "Maximum Pixels per Write" -> [w426]
              tunnel: 5000 ("Write Timeout (ms)") -> [w422]
              tunnel: w408 -> [w417]
              tunnel: [w416] -> w392
              stop <- w429 stop-if-true
              # "Copy the pixels from the image\nto the FIFO."
              # "Stop if there are no\npixels left in the \nregion or there is\nan error."
              n137 = Max & Min(x=w427, y=w426) -> (min(x,y)=w425:u32)  [unwired: 1 out]
              n138 = in-place {
                in-place-border: w425 -> [w444]
                in-place-border: [w446] -> w435
                in-place-border: w434 -> [w443]
                in-place-border: w433 -> [w441]
                in-place-border: [w442] -> w432
                in-place-border: [w438] -> w424
                in-place-border: [w437] -> w418
                w445 = u32 0  # Region Offset
                n139 = in-place-dvr #1(w436) -> (w440:u32[][], w438:errorcluster)
                n140 = while {
                  tunnel: w440 -> [w453]
                  shift-right: [w465] -> _
                  shift-left: w445 -> [w464]
                  tunnel: w444 -> [w467]
                  shift-right: [w458] -> w442
                  shift-left: w443 -> [w454]
                  shift-right: [w448] -> w437
                  shift-left: u8[] [] -> [w450]
                  shift-right: [w455] -> w446
                  shift-left: w441 -> [w451]
                  stop <- w447 stop-if-true
                  # "Stop when we run out\nof room in the current\nregion."
                  # "Reset the column offset if we copied\nall of the pixels from the current\nrow."
                  # "Move to next row if we copied\nall of the pixels from the\ncurrent row."
                  n141 = Index Array(array=w453, index (row)=w451) -> (element=w452:u32[])  [unwired: 1 in]
                  n142 = Subtract(x=w467, y=w464) -> (x-y=w466:u32)
                  n143 = Array Size(array=w452) -> (size(s)=w463:i32)
                  n144 = Subtract(x=w463, y=w454) -> (x-y=w461:u32)
                  n145 = Less Or Equal?(x=w466, y=w461) -> (x <= y?=w447:bool)
                  n146 = Select(t=w466, s=w447, f=w461) -> (s? t:f=w462:u32)
                  n147 = Add(x=w462, y=w454) -> (x+y=w459:u32)
                  n148 = Array Subset(array=w452, index=w454, length=w462) -> (w449:u32[])
                  n149 = Equal?(x=w459, y=w463) -> (x = y?=w457:bool)
                  n150 = Build Array (concatenate)(w450, w449) -> (w448:u32[])
                  n151 = Increment(x=w451) -> (x+1=w456:u32)
                  n152 = Select(t=u32 0 ("Elements In Region"), s=w457, f=w459) -> (s? t:f=w458:u32)
                  n153 = Select(t=w456, s=w457, f=w451) -> (s? t:f=w455:u32)
                  n154 = Add(x=w464, y=w462) -> (x+y=w465:u32)
                }
                n155 = in-place-dvr #1(w440) -> (w431:refnum<data-value>, w423:errorcluster)
              }
              n156 = Subtract(x=w427, y=w425) -> (x-y=w430:u32)
              n157 = Equal To 0?(x=w430) -> (x = 0?=w428:bool)
              n158 = Merge Errors(w417, w424, w423) -> (w420:errorcluster)
              n159 = xnode "Invoke Method"("FPGA VI Reference In"=w421, "error in"=w420, "Data"=w418, "Timeout (ms)"=w422) -> ("FPGA VI Reference Out"=w416:refnum<k20>, "error out"=w419:errorcluster)  [unwired: 1 out]
              n160 = Or(x=w428, y=w419) -> (x .or. y?=w429:bool)
            }
            n161 = shared-variable-write(w395, w394, w398) -> (w397:refnum<k21>, w396:errorcluster)  [unwired: 1 in, 1 out]
            n162 = Delete Data Value Reference(data value reference=w407, error in=w406) -> (error out=w399:errorcluster)  [unwired: 1 out]
          }
        }
      }
    }
    n163 = Or(x=w356, y="Stop") -> (x .or. y?=w361:bool)
  }
  n164 = Destroy Stream Endpoint(8:w53, 11:w52) -> (0:w44:errorcluster)
  n165 = Destroy Stream Endpoint(8:w83, 11:w84) -> (0:w43:errorcluster)
  n166 = Destroy Stream Endpoint(8:w64, 11:w65) -> (0:w45:errorcluster)
  n167 = Destroy Stream Endpoint(8:w101, 11:w102) -> (0:w98:errorcluster)
  n168 = Destroy Stream Endpoint(8:w87, 11:w86) -> (0:w85:errorcluster)
  n169 = Destroy Stream Endpoint(8:w67, 11:w66) -> (0:w46:errorcluster)
  n170 = Destroy Stream Endpoint(8:w76, 11:w77) -> (0:w47:errorcluster)
  n171 = Destroy Stream Endpoint(8:w106, 11:w105) -> (0:w99:errorcluster)
  n172 = Merge Errors(w99, w98, w85, w47, w46, w45, w44, w43) -> (→"error out 2":errorcluster)
  n173 = stacked-sequence {
    tunnel: w11 -> [w468]
    tunnel: [w468] -> w14
    frame #0 {
      n174 = local write "Stop"(TRUE ("Stop")) -> ()
    }
  }
  n175 = Destroy Stream Endpoint(8:w28, 11:w29) -> ()  [unwired: 1 out]
  n176 = Merge Errors(w14) -> (w15:errorcluster)
  n177 = call <vilib>:"IMAQdx Stop Acquisition.vi"("error in"=w14, "Session In"=w13) -> ("error out"=w19:errorcluster, "Session Out"=w20:T1)  [unwired: 8 in]
  n178 = xnode "Close FPGA VI Reference"("FPGA VI Reference In"=w12, "error in"=w15) -> ("error out"=w22:errorcluster)
  n179 = call <vilib>:"IMAQdx Close Camera.vi"("error in"=w19, "Session In"=w20) -> ("error out"=w18:errorcluster)  [unwired: 9 in]
  n180 = call "IMAQ Dispose"("Image"=w10, "error in (no error)"=w22) -> ("error out"=w21:errorcluster)  [unwired: 4 in]
  n181 = Merge Errors(w18, w21) -> (w17:errorcluster)
  n182 = xnode "Close FPGA VI Reference"("FPGA VI Reference In"=w9, "error in"=w17) -> ("error out"=w16:errorcluster)
  "Error Out 2" <- w16
  n183 = stacked-sequence {
    tunnel: w16 -> [_]
    frame #0 {
      n184 = local write "Stop"(FALSE ("Stop")) -> ()
    }
  }
  "RecGaussian1?" <- w1
  "RecGaussian2?" <- w1
